vi "testUpload_raw.vi"() -> ()   [LabVIEW 2025]
panel:
  out "error out 3":errorcluster
  out "error out 2":errorcluster
  out "Device":i32
  out "device 2":enum16{"CPU", "GPU0"}(ring)=enum."GPU0"
  in  "device":enum16{"CPU", "GPU0"}(ring)=enum."GPU0"
  out "loadedImgSucc":i32
  out "error out":errorcluster
  in  "PathImage":path=path "D:/Test/dllTest/images_2"
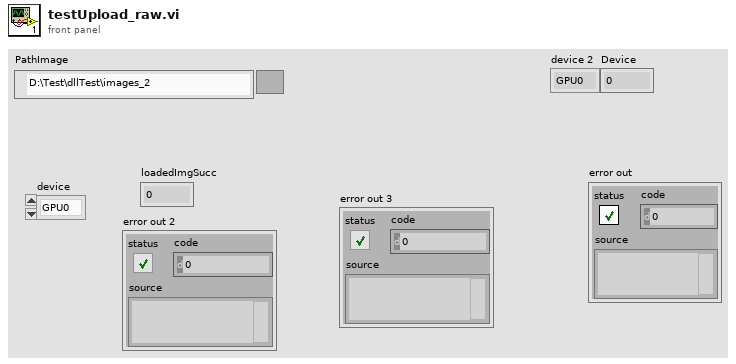
[diagram p1: front panel]
types:
  T1 = typedef "IMAQ Image.ctl" = refnum<image>
  T2 = enum32{"Map Pixel Pointer", "Unmap Pixel Pointer", "Get Pixels Infos"}
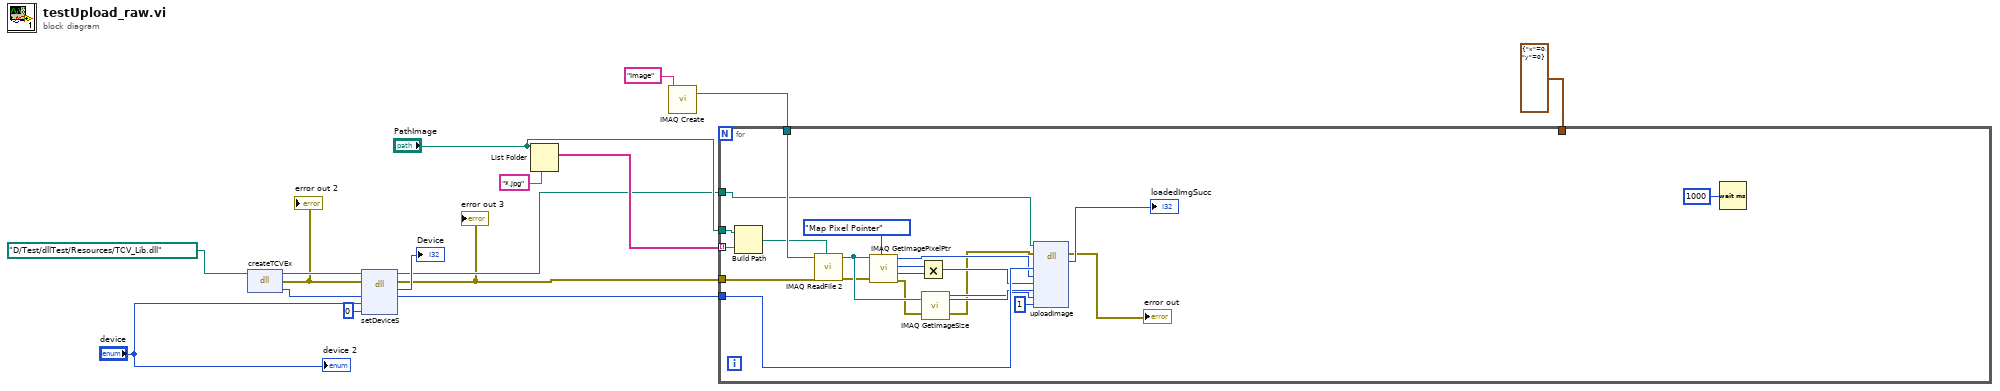
[diagram p0: block diagram]
diagram:
  n1 = dll-call lib="D:/Test/adslvPackageDev/Resources/TCV_Lib.dll" fn="createTCVEx"(path in=path "D:/Test/dllTest/Resources/TCV_Lib.dll") -> (path out=w9:path, error out=w3:errorcluster, "tcv"=w8:u64)  [unwired: 2 in]
  "error out 2" <- w3
  n2 = dll-call lib="D:/Test/dllTest/Resources/TCV_Lib.dll" fn="setDeviceS"(path in=w9, error in=w3, "tcv"=w8, "device"="device", "external"=u64 0) -> (path out=w4:path, error out=w2:errorcluster, "Device"=→"Device":i32, "tcv"=w7:u64)  [unwired: 3 in]
  "error out 3" <- w2
  n3 = List Folder(path="PathImage", pattern="*.jpg") -> (filenames=w12:string[])  [unwired: 2 in, 3 out]
  n4 = call "IMAQ Create"("Image Name"="Image") -> ("New Image"=w15:T1)  [unwired: 4 in, 1 out]
  n5 = for {
    tunnel: "PathImage" -> [w38]
    tunnel: w15 -> [w35]
    tunnel: cluster{"x":i32, "y":i32} {"x"=0, "y"=0} -> [_]
    tunnel: w12 -> [w36] mode=indexing
    tunnel: w7 -> [w27]
    tunnel: w4 -> [w28]
    tunnel: w2 -> [w21]
    n6 = Build Path(base path=w38, name or relative path=w36) -> (appended path=w34:path)
    n7 = call "IMAQ ReadFile 2"("File Path"=w34, "error in (no error)"=w21, "Image"=w35) -> ("error out"=w18:errorcluster, "Image Out"=w30:T1)  [unwired: 4 in, 3 out]
    n8 = call "IMAQ GetImagePixelPtr"("Function"=T2."Map Pixel Pointer", "error in (no error)"=w18, "Image"=w30) -> ("error out"=w17:errorcluster, "Pixel Size (Bytes)"=w32:i32, "LineWidth(Pixels)"=w31:i32, "Pixel Pointer out"=w26:u64)  [unwired: 3 in, 2 out]
    n9 = Multiply(x=w31, y=w32) -> (x*y=w25:i32)
    n10 = call "IMAQ GetImageSize"("Image"=w30, "error in (no error)"=w17) -> ("Y Resolution"=w24:i32, "X Resolution"=w23:i32, "error out"=w20:errorcluster)  [unwired: 2 in]
    n11 = dll-call lib="D:/Test/dllTest/Resources/TCV_Lib.dll" fn="uploadImage"(path in=w28, error in=w20, "tcv"=w27, "lvptr"=w26, "lw"=w25, "h"=w24, "w"=w23, "norm"=1) -> (error out=→"error out":errorcluster, "succ"=→"loadedImgSucc":i32)  [unwired: 7 in, 1 out]
    n12 = Wait (ms)(milliseconds to wait=u32 1000) -> ()  [unwired: 1 out]
  }
  "device 2" <- "device"
